vi "LabVIEW version.vi"() -> (3 "Application:Version Year with bitness":string)   [LabVIEW 2021]
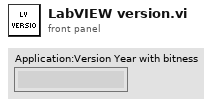
[diagram p1: front panel]
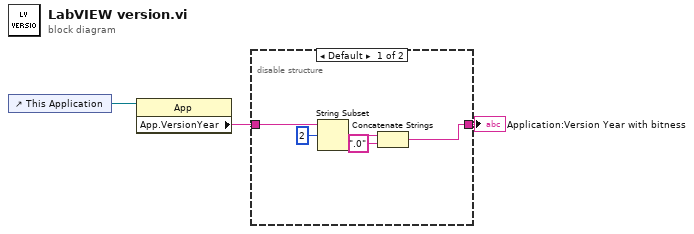
[diagram p0: block diagram]
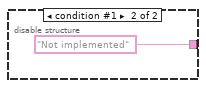
[diagram p2: hidden frame]
diagram:
  n1 = control-ref of="This Application"() -> (w3:refnum<vi>)
  n2 = property class="App"(reference=w3) -> ("App.VersionYear"=w1:string)  [unwired: 1 in, 2 out]
  n3 = disable-structure shown="Default" {
    disable-tunnel: w1 -> [w8 _]
    disable-tunnel: [w4 "Not implemented" ("App.VersionYear")] -> w2
    frame condition #0 (active) {
      n4 = String Subset(string=w8, offset (0)=2) -> (substring=w6:string)  [unwired: 1 in]
      n5 = Concatenate Strings(w6, ".0" ("string")) -> (w4:string)
    }
    frame condition #1 {
    }
  }
  "Application:Version Year with bitness" <- w2
